vi "Read Source Value.vi"(8 "error in (no error)":errorcluster, 11 "Power Supply in":refnum<class "Power Supply.lvclass">) -> (0 "error out":errorcluster, 2 "Source Value":dbl, 3 "Power Supply out":refnum<class "Power Supply.lvclass">)   [LabVIEW 2011, in "Power Supply.lvclass"]
uses:
  Power Supply.lvclass
  Power Supply.lvclass/Power Supply.ctl
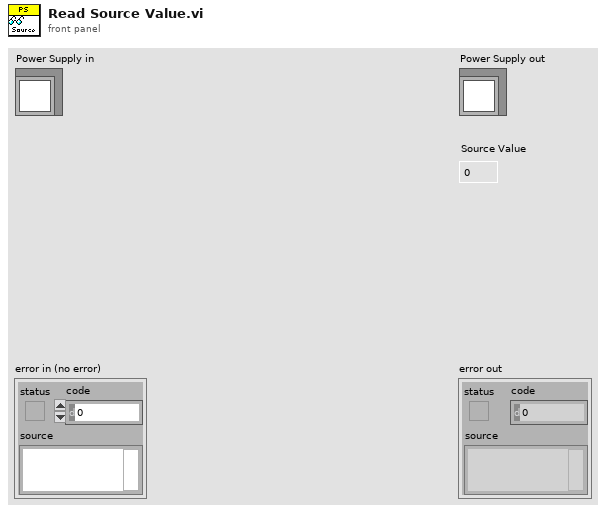
[diagram p1: front panel]
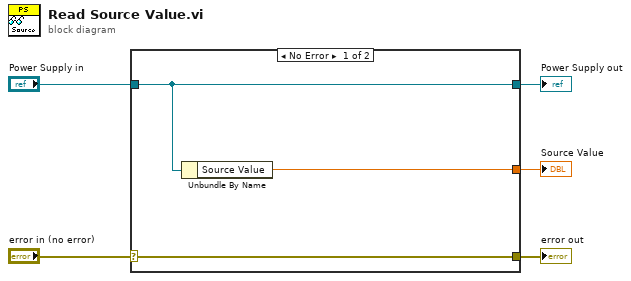
[diagram p0: block diagram]
diagram:
  n1 = case shown="No Error" "error in (no error)" {
    selector: "error in (no error)" -> [w8 w9]
    tunnel: [w8 w9] -> w4
    tunnel: [w7 w10] -> w2
    tunnel: "Power Supply in" -> [w7 w10]
    tunnel: [w6 _] -> w1
    frame No Error {
      n2 = Unbundle By Name(w7) -> ("Source Value"=w6:dbl)
    }
    frame Error {
    }
  }
  "error out" <- w4
  "Power Supply out" <- w2
  "Source Value" <- w1
